vi "OneCycleRamp1.vi"(11 "TestCycleParameters":T1={"TAmb"=20.0, "HeaterTestTemp"=-80.0, "HeaterTestDwell(min)"=30, "HeaterTestDuration"=15, "MinOpTemp"=-50.0, "MinOpDwell(min)"=30, "TestHeatingRate (deg/min)"=0.4, "SurviveCycleParameters"={"MinSurviveTemp"=-130.0, "MinSurvive Dwell(min)"=60, "MaxSurviveTemp"=50.0, "MaxSurviveDwell(min)"=30, "ControlInput"=0, "ColdStandOff"=-50.0, "HotStandoff"=0.0, "SteadyPWM"=20, "MaxCoolingRate (deg/min)"=3.75, "MaxHeatingRate (deg/min)"=2.5}, "CycleType"=0, "MaxOpTemp"=-50.0, "MinOpDwell(min)"=30} {"CycleType" items=["Survival", "Operational"]; "SurviveCycleParameters"."SteadyPWM" min=0 max=100 step=1; "SurviveCycleParameters"."ControlInput" items=["3A", "3B", "3C", "3D", "4A", "4B", "4C", "4D"]}) -> (3 "Profile":cluster{dbl[], dbl[]}(graph)={[0.0, 25.0, 85.0, 97.5, 127.5, 142.5, 150.0, 180.0, 430.0, 460.0], [20.0, -130.0, -130.0, -80.0, -80.0, -80.0, -50.0, -50.0, 50.0, 50.0]})   [LabVIEW 2024]
uses:
  controls/TestCycleParams.ctl
  controls/SurviveCycleParams.ctl
  controls/ControlInput.ctl
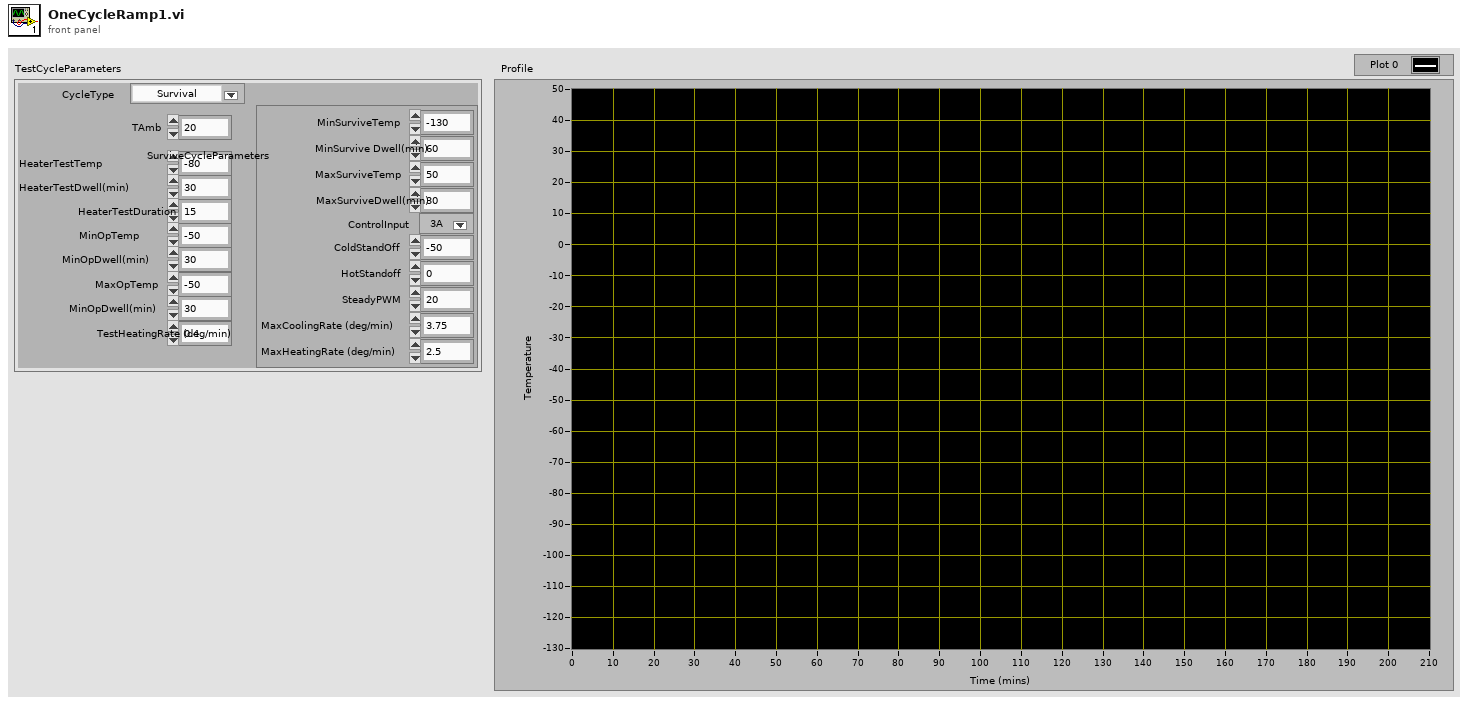
[diagram p1: front panel]
types:
  T1 = typedef "TestCycleParams.ctl" = cluster{"TAmb":dbl, "HeaterTestTemp":dbl, "HeaterTestDwell(min)":i32, "HeaterTestDuration":i32, "MinOpTemp":dbl, "MinOpDwell(min)":i32, "TestHeatingRate (deg/min)":dbl, "SurviveCycleParameters":T2, "CycleType":u16, "MaxOpTemp":dbl, "MinOpDwell(min)":i32}
  T2 = typedef "SurviveCycleParams.ctl" = cluster{"MinSurviveTemp":dbl, "MinSurvive Dwell(min)":i32, "MaxSurviveTemp":dbl, "MaxSurviveDwell(min)":i32, "ControlInput":T3, "ColdStandOff":dbl, "HotStandoff":dbl, "SteadyPWM":i32, "MaxCoolingRate (deg/min)":dbl, "MaxHeatingRate (deg/min)":dbl}
  T3 = typedef "ControlInput.ctl" = u16
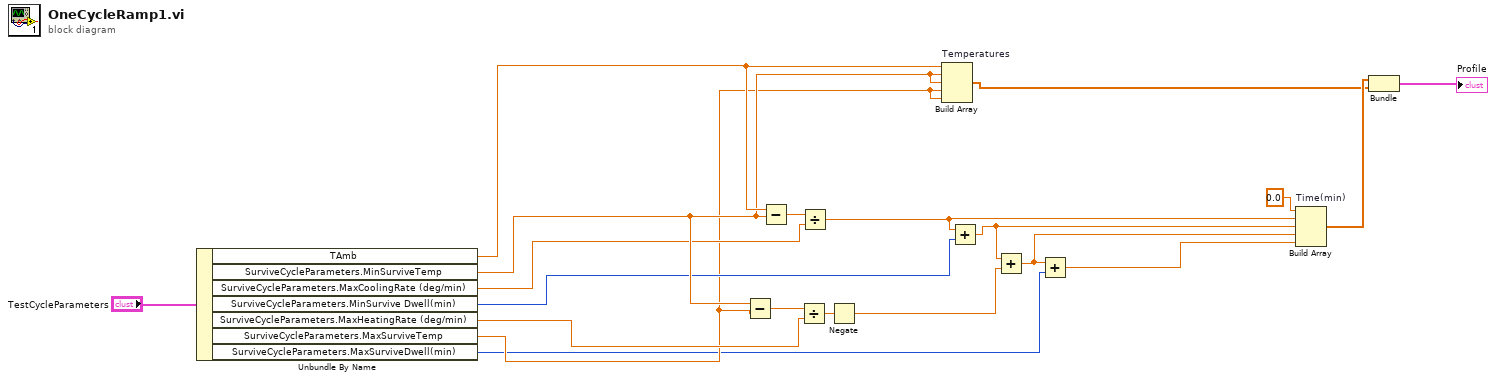
[diagram p0: block diagram]
diagram:
  n1 = Unbundle By Name("TestCycleParameters") -> ("TAmb"=w9:dbl, "SurviveCycleParameters.MinSurviveTemp"=w8:dbl, "SurviveCycleParameters.MaxCoolingRate (deg/min)"=w7:dbl, "SurviveCycleParameters.MinSurvive Dwell(min)"=w6:i32, "SurviveCycleParameters.MaxHeatingRate (deg/min)"=w5:dbl, "SurviveCycleParameters.MaxSurviveTemp"=w4:dbl, "SurviveCycleParameters.MaxSurviveDwell(min)"=w2:i32)
  n2 = Subtract(x=w8, y=w4) -> (x-y=w14:dbl)
  n3 = Subtract(x=w9, y=w8) -> (x-y=w19:dbl)
  n4 = Divide(x=w14, y=w5) -> (x/y=w13:dbl)
  n5 = Divide(x=w19, y=w7) -> (x/y=w18:dbl)
  n6 = Negate(x=w13) -> (-x=w11:dbl)
  n7 = Build Array "Temperatures"(w9, w8, w8, w4, w4) -> (w16:dbl[])
  n8 = Add(x=w18, y=w6) -> (x+y=w12:dbl)
  n9 = Add(x=w12, y=w11) -> (x+y=w3:dbl)
  n10 = Add(x=w3, y=w2) -> (x+y=w1:dbl)
  n11 = Build Array "Time(min)"(0.0, w18, w12, w3, w1) -> (w17:dbl[])
  n12 = Bundle(w17, w16) -> (→"Profile":cluster{dbl[], dbl[]})  [unwired: 1 in]
